vi "practice07_lcd_message.vi"() -> ()   [LabVIEW 2025]
uses:
  <vilib>/Instr/_visa.llb/VISA Configure Serial Port (Instr).vi
panel:
  in  "Mensaje enviado":string
  in  "stop":bool
  out "Mensaje leido":string
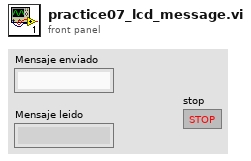
[diagram p1: front panel]
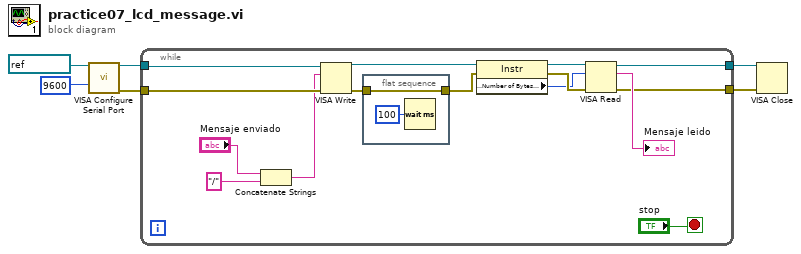
[diagram p0: block diagram]
diagram:
  n1 = call-poly "VISA Configure Serial Port"("VISA resource name"=refnum<visa-resource-name> "COM3", "parity (0:none)"=9600) -> ("VISA resource name out"=w4:refnum<visa-resource-name>, "error out"=w3:errorcluster)  [unwired: 12 in]
  n2 = while {
    tunnel: w4 -> [w18]
    tunnel: w3 -> [w17]
    tunnel: [w11] -> w2
    tunnel: [w10] -> w1
    stop <- "stop" stop-if-true
    n3 = Concatenate Strings("Mensaje enviado", "/" ("string")) -> (w9:string)
    n4 = VISA Write(VISA resource name=w18, write buffer=w9, error in (no error)=w17) -> (VISA resource name out=w16:refnum<visa-resource-name>, error out=w15:errorcluster)  [unwired: 1 out]
    n5 = flat-sequence {
      tunnel: w15 -> [w23]
      tunnel: [w23] -> w14
      frame #0 {
        n6 = Wait (ms)(milliseconds to wait=u32 100) -> ()  [unwired: 1 out]
      }
    }
    n7 = property class="Instr"(reference=w16, error in=w14) -> (reference out=w20:refnum<visa-resource-name>, error out=w19:errorcluster, "Serial Settings:Number of Bytes at Serial Port"=w13:u32)
    n8 = VISA Read(VISA resource name=w20, byte count=w13, error in (no error)=w19) -> (VISA resource name out=w11:refnum<visa-resource-name>, read buffer=→"Mensaje leido":string, error out=w10:errorcluster)  [unwired: 1 out]
  }
  n9 = VISA Close(VISA resource name=w2, error in (no error)=w1) -> ()  [unwired: 1 out]
